vi "Calc - TUEG.vi"(11 "01-00-9213":dbl[](array[numeric])) -> (1 "TUEGDelta":dbl, 2 "TUEGLower":dbl, 3 "TUEGUpper":dbl)   [LabVIEW 2018, in "Controller (Host).lvlib"]
uses:
  Controller (Host).lvlib
  <vilib>/Analysis/baseanly.llb/Mean (DBL).vi
  <vilib>/Analysis/NI_AALBase.lvlib
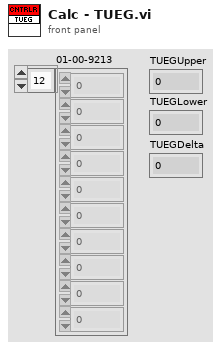
[diagram p1: front panel]
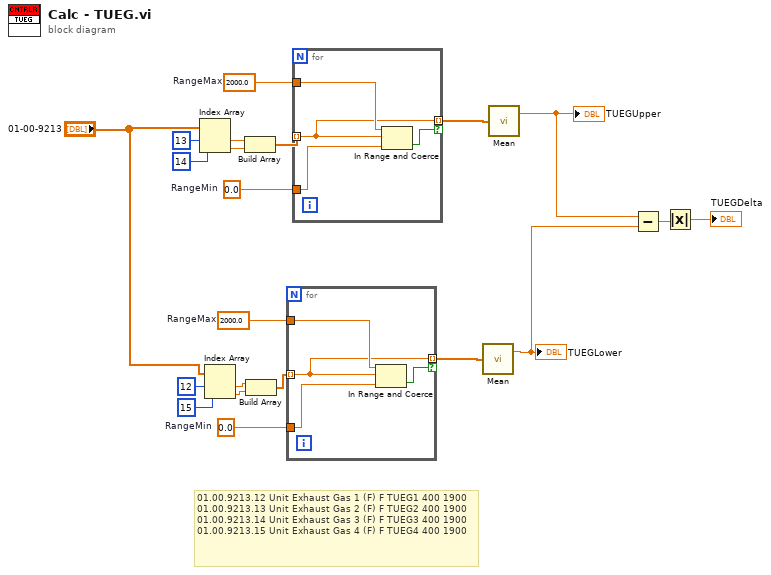
[diagram p0: block diagram]
diagram:
  w17 = 2000.0  # RangeMax
  w16 = 0.0  # RangeMin
  w20 = 2000.0  # RangeMax
  w21 = 0.0  # RangeMin
  # "01.00.9213.12\tUnit Exhaust Gas 1 (F)\tF\tTUEG1\t400\t1900\n01.00.9213.13\tUnit Exhaust Gas 2 (F)\tF\tTUEG2\t400\t1900\n01.00.9213.14\tUnit Exhaust Gas 3 (F)\tF\tTUEG3\t400\t1900\n01.00.9213.15\tUnit Exhaust Gas 4 (F)\tF\tTUEG4\t400\t1900"
  n1 = Index Array(array="01-00-9213", index #1=13 ("index"), index #2=14 ("index")) -> (element #1=w9:dbl, element #2=w8:dbl)
  n2 = Index Array(array="01-00-9213", index #1=12 ("index"), index #2=15 ("index")) -> (element #1=w7:dbl, element #2=w6:dbl)
  n3 = Build Array(w9, w8) -> (w10:dbl[])
  n4 = Build Array(w7, w6) -> (w5:dbl[])
  n5 = for {
    tunnel: w5 -> [w23] mode=indexing
    tunnel: w16 -> [w24]
    tunnel: w17 -> [w25]
    tunnel: [w23] -> w18 mode=indexing if=w22
    n6 = In Range and Coerce(upper limit=w25, x=w23, lower limit=w24) -> (In Range?=w22:bool)  [unwired: 1 out]
  }
  n7 = for {
    tunnel: w10 -> [w27] mode=indexing
    tunnel: w21 -> [w28]
    tunnel: w20 -> [w29]
    tunnel: [w27] -> w19 mode=indexing if=w26
    n8 = In Range and Coerce(upper limit=w29, x=w27, lower limit=w28) -> (In Range?=w26:bool)  [unwired: 1 out]
  }
  n9 = call-poly <vilib>:"Mean.vi"("X"=w18) -> ("mean"=w3:dbl)  [unwired: 1 out]
  "TUEGLower" <- w3
  n10 = call-poly <vilib>:"Mean.vi"("X"=w19) -> ("mean"=w4:dbl)  [unwired: 1 out]
  "TUEGUpper" <- w4
  n11 = Subtract(x=w4, y=w3) -> (x-y=w2:dbl)
  n12 = Absolute Value(x=w2) -> (abs(x)=→"TUEGDelta":dbl)
